vi "index-trigger-TEST.vi"() -> ()   [LabVIEW 2015]
panel:
  out "Array 2":bool[](array[boolean])
  in  "Array":i16[](array[numeric])
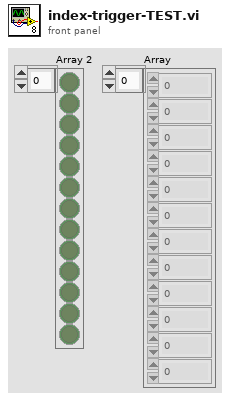
[diagram p1: front panel]
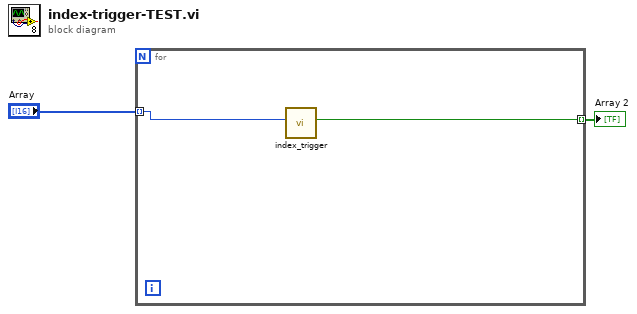
[diagram p0: block diagram]
diagram:
  n1 = for {
    tunnel: "Array" -> [w4] mode=indexing
    tunnel: [w3] -> w2 mode=indexing
    n2 = call "index_trigger.vi"("fifo-counter"=w4) -> ("index trigger"=w3:bool)  [unwired: 10 in]
  }
  "Array 2" <- w2
